vi "Get Default Configuration Parameters.vi"() -> (0 "Default Config Params":variant)   [LabVIEW 2023, in "AMS Climate Chamber Template.lvlib" / "AMS Climate Chamber Template.lvclass"]
uses:
  AMS Climate Chamber Template.lvclass
  Configuration Params.ctl
  <vilib>/ADAS Replay HIL/Template Node/Plugin/Template Node/Common Configuration Params.ctl
  <vilib>/ADAS Replay HIL/Template Node/Plugin/Template Node/Template Node.lvclass
panel:
  # "Set default parameters on the block diagram."
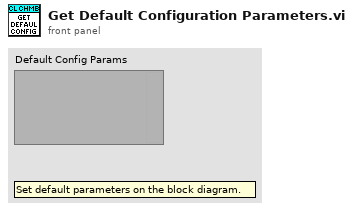
[diagram p1: front panel]
types:
  T1 = typedef "AMS Climate Chamber Template.lvlib/AMS Climate Chamber Template.lvclass/Configuration Params.ctl" = cluster{"Common":T2, "Amount of Channels":u32, "Address":string}
  T2 = typedef "Template Node.lvlib/Template Node.lvclass/Common Configuration Params.ctl" = cluster{"Iteration Interval (s)":dbl, "T0 (ns)":u64, "Priority":i32, "Processor":i32, "Wait in Ready State":bool}
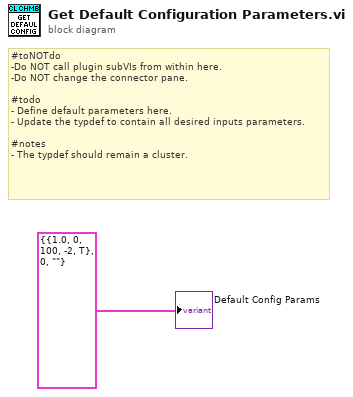
[diagram p0: block diagram]
diagram:
  # "#toNOTdo\n-Do NOT call plugin subVIs from within here.\n-Do NOT change the connector pane.\n\n#todo\n- Define default parameters here.\n- Update the typdef to contain all desired inputs parameters.\n\n#notes\n- The typdef should remain a cluster."
  "Default Config Params" <- T1 {"Common"={"Iteration Interval (s)"=1.0, "T0 (ns)"=0, "Priority"=100, "Processor"=-2, "Wait in Ready State"=TRUE}, "Amount of Channels"=0, "Address"=""} ("Default Parameters")
